vi "AlliGator Find Cursor Connecting Line Intersection(s) with Universal Circle.vi"(8 "Error In":errorcluster, 11 "XY Graph Refnum":refnum<vi>) -> (0 "Error Out":errorcluster, 2 "Intersection 2":cluster{"x":dbl, "y":dbl}, 3 "Intersection 1":cluster{"x":dbl, "y":dbl})   [LabVIEW 2021, in "AlliGator Phasor Graph.lvlib"]
doc: "Computes intersections of a segment connecting the first two cursors of the Phasor Graph with the universal circle."
uses:
  AlliGator Phasor Graph.lvlib
  Math/Math.lvlib
panel:
  # "see the AlliGator License on the block diagram (Ctrl+E or Window:Show Block Diagram)"
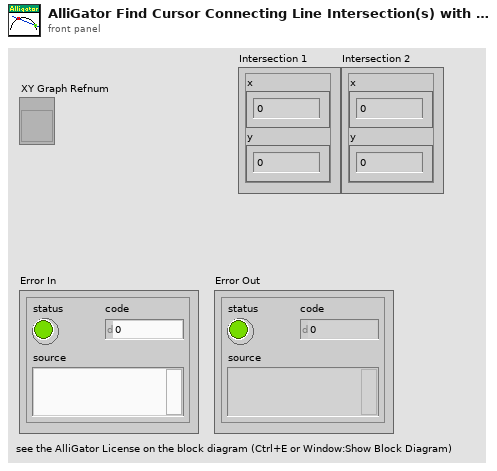
[diagram p1: front panel]
types:
  T1 = typedef "LVCursorListTypeDef.ctl" = cluster{"Name":string, "Color":u32, "Style":u8, "Point Style":u8, "Name Visible":bool, "Allow Drag":bool, "Cursor Mode":u32, "Plot":i32, "Index":i32, "Position":cluster{"X":dbl, "Y":dbl}, "X Scale":u32, "Y Scale":u32, "Watch Plots":i32[], "Watch All Plots":bool, "Plot Area":i32, "Label Offset":cluster{"X":dbl, "Y":dbl}}[]
  T2 = cluster{"Name":string, "Color":u32, "Style":u8, "Point Style":u8, "Name Visible":bool, "Allow Drag":bool, "Cursor Mode":u32, "Plot":i32, "Index":i32, "Position":cluster{"X":dbl, "Y":dbl}, "X Scale":u32, "Y Scale":u32, "Watch Plots":i32[], "Watch All Plots":bool, "Plot Area":i32, "Label Offset":cluster{"X":dbl, "Y":dbl}}
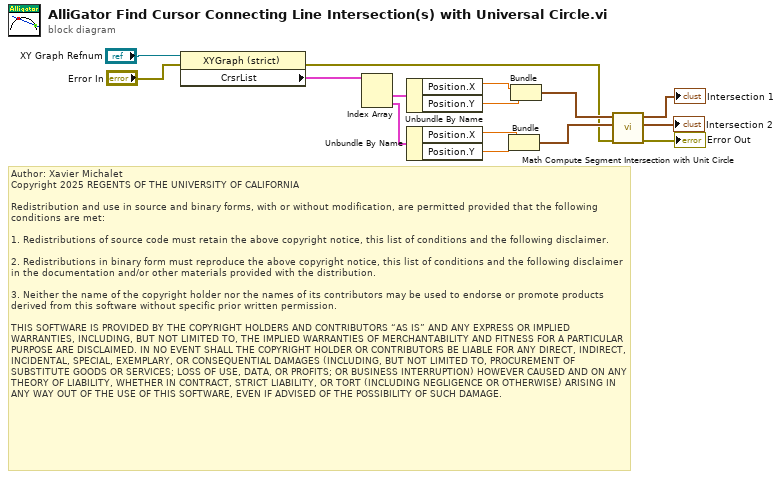
[diagram p0: block diagram]
diagram:
  # "Author: Xavier Michalet\nCopyright 2025 REGENTS OF THE UNIVERSITY OF CALIFORNIA\n\nRedistribution and use in source and binary forms, with or without modification, are permitted provided that the following conditions are met:\n\n1. Redistributions of source code must retain the above copyright notice, this list of conditions and the following disclaimer.\n\n2. Redistributions in binary form must reproduce the above copyright notice, this list of conditions and the following disclaimer in the documentation and/or other materials provided with the distribution.\n\n3. Neither the name of the copyright holder nor the names of its contributors may be used to endorse or promote products derived from this software without specific prior written permission.\n\nTHIS SOFTWARE IS PROVIDED BY THE COPYRIGHT HOLDERS AND CONTRIBUTORS “AS IS” AND ANY EXPRESS OR IMPLIED WARRANTIES, INCLUDING, BUT NOT LIMITED TO, THE IMPLIED WARRANTIES OF MERCHANTABILITY AND FITNESS FOR A PARTICULAR PURPOSE ARE DISCLAIMED. IN NO EVENT SHALL THE COPYRIGHT HOLDER OR CONTRIBUTORS BE LIABLE FOR ANY DIRECT, INDIRECT, INCIDENTAL, SPECIAL, EXEMPLARY, OR CONSEQUENTIAL DAMAGES (INCLUDING, BUT NOT LIMITED TO, PROCUREMENT OF SUBSTITUTE GOODS OR SERVICES; LOSS OF USE, DATA, OR PROFITS; OR BUSINESS INTERRUPTION) HOWEVER CAUSED AND ON ANY THEORY OF LIABILITY, WHETHER IN CONTRACT, STRICT LIABILITY, OR TORT (INCLUDING NEGLIGENCE OR OTHERWISE) ARISING IN ANY WAY OUT OF THE USE OF THIS SOFTWARE, EVEN IF ADVISED OF THE POSSIBILITY OF SUCH DAMAGE."
  n1 = property class="XYGraph (strict)"(reference="XY Graph Refnum", error in="Error In") -> (error out=w2:errorcluster, "CrsrList"=w11:T1)  [unwired: 1 out]
  n2 = Index Array(array=w11) -> (element #1=w13:T2, element #2=w12:T2)  [unwired: 2 in]
  n3 = Unbundle By Name(w13) -> ("Position.X"=w7:dbl, "Position.Y"=w6:dbl)
  n4 = Unbundle By Name(w12) -> ("Position.X"=w4:dbl, "Position.Y"=w3:dbl)
  n5 = Bundle("X"=w4, "Y"=w3) -> (w5:cluster{"X":dbl, "Y":dbl})  [unwired: 1 in]
  n6 = Bundle("X"=w7, "Y"=w6) -> (w8:cluster{"X":dbl, "Y":dbl})  [unwired: 1 in]
  n7 = call "Math Compute Segment Intersection with Unit Circle.vi"("Error In"=w2, "Point 2"=w5, "Point 1"=w8) -> ("Error Out"=→"Error Out":errorcluster, "Intersection 2"=→"Intersection 2":cluster{"x1m":dbl, "y1m":dbl}, "Intersection 1"=→"Intersection 1":cluster{"x1p":dbl, "y1p":dbl})  [unwired: 6 in]
